vi "ParseTXT.vi"(8 "error in (no error)":errorcluster, 10 "Path":path=path "C:/LVLibrary/XNET/XCP_DaqDtoID/XCP_DaqDtoId/ECUMCLog/XCP or CCP Master_Protocol_Log.txt", 11 "DAQList in":refnum<class "DAQList.lvclass">) -> (0 "error out":errorcluster, 2 "CAN Frames":T1[](array[typedef])=[{"timestamp"=timestamp(0 s since 1904-01-01), "payload"=[255, 0, 109, 101, 0, 39, 0, 0, 0], "identifier"=1996, "type"=0, "extended?"=FALSE, "echo?"=FALSE}, {"timestamp"=timestamp(0 s since 1904-01-01), "payload"=[253, 255, 255, 255, 0, 0, 0, 0, 0], "identifier"=1996, "type"=0, "extended?"=FALSE, "echo?"=FALSE}, {"timestamp"=timestamp(0 s since 1904-01-01), "payload"=[251, 255, 255, 255, 0, 0, 0, 0, 0], "identifier"=1996, "type"=0, "extended?"=FALSE, "echo?"=FALSE}, {"timestamp"=timestamp(0 s since 1904-01-01), "payload"=[218, 120, 84, 83, 83, 0, 0, 0, 0], "identifier"=1996, "type"=0, "extended?"=FALSE, "echo?"=FALSE}, {"timestamp"=timestamp(0 s since 1904-01-01), "payload"=[215, 0, 0, 0, 66, 0, 0, 0, 0], "identifier"=1996, "type"=0, "extended?"=FALSE, "echo?"=FALSE}, {"timestamp"=timestamp(0 s since 1904-01-01), "payload"=[245, 7, 114, 76, 101, 110, 0, 0, 0], "identifier"=1996, "type"=0, "extended?"=FALSE, "echo?"=FALSE}, {"timestamp"=timestamp(0 s since 1904-01-01), "payload"=[245, 7, 114, 76, 101, 110, 0, 0, 0], "identifier"=1996, "type"=0, "extended?"=FALSE, "echo?"=FALSE}, {"timestamp"=timestamp(0 s since 1904-01-01), "payload"=[245, 5, 114, 76, 101, 110, 0, 0, 0], "identifier"=1996, "type"=0, "extended?"=FALSE, "echo?"=FALSE}, {"timestamp"=timestamp(0 s since 1904-01-01), "payload"=[215, 0, 0, 0, 0, 0, 0, 0, 0], "identifier"=1996, "type"=0, "extended?"=FALSE, "echo?"=FALSE}, {"timestamp"=timestamp(0 s since 1904-01-01), "payload"=[245, 7, 66, 105, 116, 0, 0, 0, 0], "identifier"=1996, "type"=0, "extended?"=FALSE, "echo?"=FALSE}, {"timestamp"=timestamp(0 s since 1904-01-01), "payload"=[245, 7, 66, 105, 116, 0, 0, 0, 0], "identifier"=1996, "type"=0, "extended?"=FALSE, "echo?"=FALSE}, {"timestamp"=timestamp(0 s since 1904-01-01), "payload"=[245, 5, 66, 105, 116, 0, 0, 0, 0], "identifier"=1996, "type"=0, "extended?"=FALSE, "echo?"=FALSE}, {"timestamp"=timestamp(0 s since 1904-01-01), "payload"=[215, 0, 1, 0, 101, 0, 0, 0, 0], "identifier"=1996, "type"=0, "extended?"=FALSE, "echo?"=FALSE}, {"timestamp"=timestamp(0 s since 1904-01-01), "payload"=[245, 7, 114, 105, 103, 115, 0, 0, 0], "identifier"=1996, "type"=0, "extended?"=FALSE, "echo?"=FALSE}, {"timestamp"=timestamp(0 s since 1904-01-01), "payload"=[245, 7, 114, 105, 103, 115, 0, 0, 0], "identifier"=1996, "type"=0, "extended?"=FALSE, "echo?"=FALSE}, {"timestamp"=timestamp(0 s since 1904-01-01), "payload"=[245, 6, 114, 105, 103, 115, 0, 0, 0], "identifier"=1996, "type"=0, "extended?"=FALSE, "echo?"=FALSE}, {"timestamp"=timestamp(0 s since 1904-01-01), "payload"=[215, 0, 2, 0, 109, 101, 0, 0, 0], "identifier"=1996, "type"=0, "extended?"=FALSE, "echo?"=FALSE}, {"timestamp"=timestamp(0 s since 1904-01-01), "payload"=[245, 7, 0, 0, 66, 0, 0, 0, 0], "identifier"=1996, "type"=0, "extended?"=FALSE, "echo?"=FALSE}, {"timestamp"=timestamp(0 s since 1904-01-01), "payload"=[245, 7, 0, 0, 66, 0, 0, 0, 0], "identifier"=1996, "type"=0, "extended?"=FALSE, "echo?"=FALSE}, {"timestamp"=timestamp(0 s since 1904-01-01), "payload"=[245, 6, 0, 0, 66, 0, 0, 0, 0], "identifier"=1996, "type"=0, "extended?"=FALSE, "echo?"=FALSE}, {"timestamp"=timestamp(0 s since 1904-01-01), "payload"=[215, 0, 3, 0, 0, 39, 0, 0, 0], "identifier"=1996, "type"=0, "extended?"=FALSE, "echo?"=FALSE}, {"timestamp"=timestamp(0 s since 1904-01-01), "payload"=[245, 7, 84, 83, 83, 0, 0, 0, 0], "identifier"=1996, "type"=0, "extended?"=FALSE, "echo?"=FALSE}, {"timestamp"=timestamp(0 s since 1904-01-01), "payload"=[245, 7, 84, 83, 83, 0, 0, 0, 0], "identifier"=1996, "type"=0, "extended?"=FALSE, "echo?"=FALSE}, {"timestamp"=timestamp(0 s since 1904-01-01), "payload"=[245, 7, 84, 83, 83, 0, 0, 0, 0], "identifier"=1996, "type"=0, "extended?"=FALSE, "echo?"=FALSE}, {"timestamp"=timestamp(0 s since 1904-01-01), "payload"=[215, 0, 4, 0, 66, 0, 0, 0, 0], "identifier"=1996, "type"=0, "extended?"=FALSE, "echo?"=FALSE}, {"timestamp"=timestamp(0 s since 1904-01-01), "payload"=[245, 7, 67, 121, 99, 108, 101, 0, 0], "identifier"=1996, "type"=0, "extended?"=FALSE, "echo?"=FALSE}, {"timestamp"=timestamp(0 s since 1904-01-01), "payload"=[245, 7, 67, 121, 99, 108, 101, 0, 0], "identifier"=1996, "type"=0, "extended?"=FALSE, "echo?"=FALSE}, {"timestamp"=timestamp(0 s since 1904-01-01), "payload"=[245, 7, 67, 121, 99, 108, 101, 0, 0], "identifier"=1996, "type"=0, "extended?"=FALSE, "echo?"=FALSE}, {"timestamp"=timestamp(0 s since 1904-01-01), "payload"=[245, 1, 67, 121, 99, 108, 101, 0, 0], "identifier"=1996, "type"=0, "extended?"=FALSE, "echo?"=FALSE}, {"timestamp"=timestamp(0 s since 1904-01-01), "payload"=[217, 255, 255, 255, 0, 0, 0, 0, 0], "identifier"=1996, "type"=0, "extended?"=FALSE, "echo?"=FALSE}, {"timestamp"=timestamp(0 s since 1904-01-01), "payload"=[233, 255, 255, 255, 0, 0, 0, 0, 0], "identifier"=1996, "type"=0, "extended?"=FALSE, "echo?"=FALSE}, {"timestamp"=timestamp(0 s since 1904-01-01), "payload"=[232, 0, 0, 0, 0, 108, 101, 0, 0], "identifier"=1996, "type"=0, "extended?"=FALSE, "echo?"=FALSE}, {"timestamp"=timestamp(0 s since 1904-01-01), "payload"=[232, 0, 0, 1, 0, 108, 101, 0, 0], "identifier"=1996, "type"=0, "extended?"=FALSE, "echo?"=FALSE}, {"timestamp"=timestamp(0 s since 1904-01-01), "payload"=[232, 1, 0, 1, 0, 108, 101, 0, 0], "identifier"=1996, "type"=0, "extended?"=FALSE, "echo?"=FALSE}, {"timestamp"=timestamp(0 s since 1904-01-01), "payload"=[231, 0, 0, 0, 101, 0, 0, 0, 0], "identifier"=1996, "type"=0, "extended?"=FALSE, "echo?"=FALSE}, {"timestamp"=timestamp(0 s since 1904-01-01), "payload"=[206, 255, 255, 255, 0, 0, 0, 0, 0], "identifier"=1996, "type"=0, "extended?"=FALSE, "echo?"=FALSE}, {"timestamp"=timestamp(0 s since 1904-01-01), "payload"=[227, 0, 0, 0, 0, 2, 0, 0, 0], "identifier"=1996, "type"=0, "extended?"=FALSE, "echo?"=FALSE}, {"timestamp"=timestamp(0 s since 1904-01-01), "payload"=[226, 0, 0, 0, 0, 0, 0, 0, 0], "identifier"=1996, "type"=0, "extended?"=FALSE, "echo?"=FALSE}, {"timestamp"=timestamp(0 s since 1904-01-01), "payload"=[225, 255, 1, 0, 112, 172, 0, 80, 0], "identifier"=1996, "type"=0, "extended?"=FALSE, "echo?"=FALSE}, {"timestamp"=timestamp(0 s since 1904-01-01), "payload"=[225, 255, 1, 0, 113, 172, 0, 80, 0], "identifier"=1996, "type"=0, "extended?"=FALSE, "echo?"=FALSE}, {"timestamp"=timestamp(0 s since 1904-01-01), "payload"=[225, 255, 1, 0, 114, 172, 0, 80, 0], "identifier"=1996, "type"=0, "extended?"=FALSE, "echo?"=FALSE}, {"timestamp"=timestamp(0 s since 1904-01-01), "payload"=[225, 255, 1, 0, 115, 172, 0, 80, 0], "identifier"=1996, "type"=0, "extended?"=FALSE, "echo?"=FALSE}, {"timestamp"=timestamp(0 s since 1904-01-01), "payload"=[224, 0, 0, 0, 0, 0, 1, 0, 0], "identifier"=1996, "type"=0, "extended?"=FALSE, "echo?"=FALSE}, {"timestamp"=timestamp(0 s since 1904-01-01), "payload"=[222, 2, 0, 0, 0, 39, 0, 0, 0], "identifier"=1996, "type"=0, "extended?"=FALSE, "echo?"=FALSE}, {"timestamp"=timestamp(0 s since 1904-01-01), "payload"=[254, 54, 78, 51, 35, 2, 0, 0, 0], "identifier"=1996, "type"=0, "extended?"=FALSE, "echo?"=FALSE}] {"payload" format="%x"; "timestamp" format="%<%.7X\n%x>T"; "type" items=["CAN Data"=0, "CAN Remote"=1, "CAN Bus Error"=2, "CAN 2.0 Data"=8, "CAN FD Data"=16, "CAN FD+BRS Data"=24, "J1939 Data"=192, "Delay"=224, "Log Trigger"=225, "Start Trigger"=226]; "identifier" format="%x"}, 3 "DAQList out":refnum<class "DAQList.lvclass">)   [LabVIEW 2019, in "XCP_DaqDtoId.lvlib" / "DAQList.lvclass"]
uses:
  DAQList.lvclass
  <vilib>/xnet/xnet.llb/XNET Frame CAN.ctl
  <vilib>/xnet/xnet.llb/XNET Frame Type CAN.ctl
  DAQList.lvclass/DAQList.ctl
  <vilib>/Utility/file.llb/Read Delimited Spreadsheet (string).vi
  <vilib>/ECUMC/ECUMC.llb/MC Get Prop XCP CRO Id.vi
  <vilib>/ECUMC/ECUMC.llb/MC Get Prop XCP DTO Id.vi
  <vilib>/ECUMC/ECUMC.lvlib
panel:
  in  "Debug Mode":bool
  in  "IDs (debug only)":u32[](array[numeric]) format="%.0x"
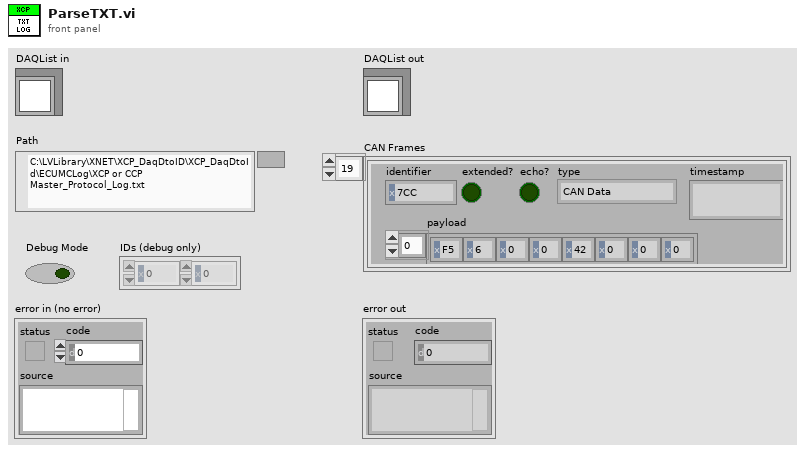
[diagram p1: front panel]
types:
  T1 = typedef "XNET Frame CAN.ctl" = cluster{"timestamp":timestamp, "payload":u8[], "identifier":u32, "type":T2, "extended?":bool, "echo?":bool}
  T2 = typedef "XNET Frame Type CAN.ctl" = u8
  T3 = typedef "ECUMC.lvlib/MC Reference.ctt" = u32
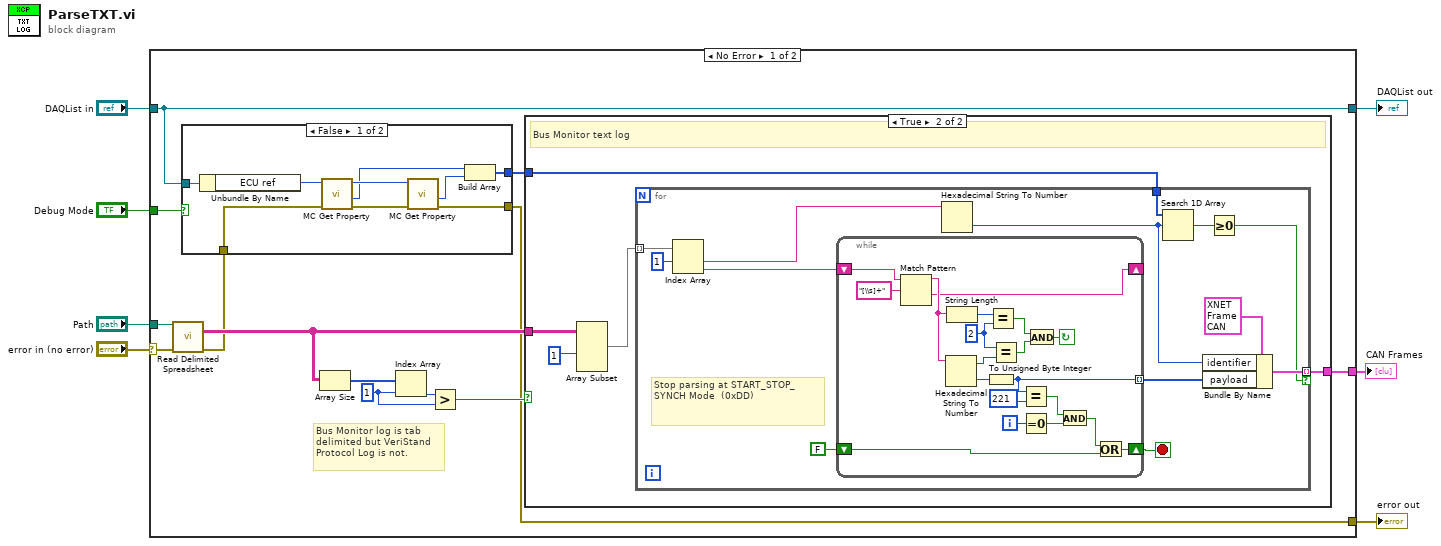
[diagram p0: block diagram]
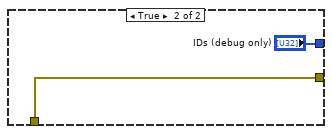
[diagram p2: hidden frame]
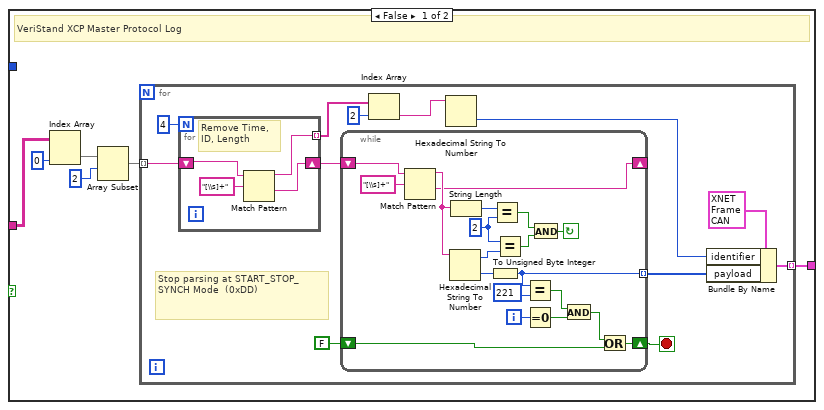
[diagram p3: hidden frame]
diagram:
  n1 = case shown="No Error" "error in (no error)" {
    selector: "error in (no error)" -> [w19 w111]
    tunnel: [w10 w111] -> w6
    tunnel: [w12 w110] -> w4
    tunnel: "DAQList in" -> [w12 w110]
    tunnel: "Path" -> [w20 _]
    tunnel: [w18 _] -> w2
    tunnel: "Debug Mode" -> [w8 _]
    frame No Error {
      w14 = 1 ("index")
      # "Bus Monitor log is tab delimited but VeriStand Protocol Log is not."
      n2 = call-poly <vilib>:"Read Delimited Spreadsheet.vi"("file path (dialog if empty)"=w20, "error in (no error)"=w19) -> ("all rows"=w17:string[][], "error out"=w11:errorcluster)  [unwired: 8 in, 4 out]
      n3 = case shown="False" w8 {
        tunnel: w12 -> [w29 _]
        tunnel: w11 -> [w27 w31]
        tunnel: [w24 w31] -> w10
        tunnel: [w21 "IDs (debug only)"] -> w9
        frame False {
          n4 = Unbundle By Name(w29) -> ("ECU ref"=w28:T3)
          n5 = call-poly <vilib>:"MC Get Property.vi"("error in"=w27, "reference in"=w28) -> ("error out"=w25:errorcluster, "XCP CRO id"=w23:u32, "reference out"=w26:T3)  [unwired: 7 in]
          n6 = call-poly <vilib>:"MC Get Property.vi"("error in"=w25, "reference in"=w26) -> ("error out"=w24:errorcluster, "XCP DTO id"=w22:u32)  [unwired: 7 in, 1 out]
          n7 = Build Array(w23, w22) -> (w21:u32[])
        }
        frame True {
        }
      }
      n8 = Array Size(array=w17) -> (size(s)=w16:i32[])
      n9 = Index Array(array=w16, index=w14) -> (element=w15:i32)
      n10 = Greater?(x=w15, y=w14) -> (0:w13:bool)
      n11 = case shown="True" w13 {
        tunnel: [w33 w74] -> w18
        tunnel: w17 -> [w32 w75]
        tunnel: w9 -> [_ w73]
        frame False {
          # "VeriStand XCP Master Protocol Log"
          n12 = Index Array(array=w32, index (col)=0 ("disabled index (col)")) -> (element=w35:string[])  [unwired: 1 in]
          n13 = Array Subset(array=w35, index=2) -> (w34:string[])  [unwired: 1 in]
          n14 = for {
            tunnel: w34 -> [w45] mode=indexing
            tunnel: [w44] -> w33 mode=indexing
            stop <- w38 stop-if-true
            # "Stop parsing at START_STOP_SYNCH Mode  (0xDD)"
            n15 = for {
              N: 4 -> [_]
              shift-right: [w70] -> w48
              shift-left: w45 -> [w72]
              tunnel: [w69] -> w43 mode=indexing
              # "Remove Time, ID, Length"
              n16 = Match Pattern(string=w72, regular expression="[\\s]+") -> (before substring=w69:string, after substring=w70:string)  [unwired: 1 in, 2 out]
            }
            n17 = while {
              shift-right: [w59] -> _
              shift-left: w48 -> [w68]
              tunnel: [w56] -> w46 mode=indexing
              shift-right: [w51] -> w38
              shift-left: FALSE -> [w50]
              i -> [w57]
              stop <- w60 continue-if-true
              w64 = 2 ("y")
              n18 = Match Pattern(string=w68, regular expression="[\\s]+") -> (before substring=w65:string, after substring=w59:string)  [unwired: 1 in, 2 out]
              n19 = Hexadecimal String To Number(string=w65) -> (offset past number=w63:i32, number=w58:u32)  [unwired: 2 in]
              n20 = String Length(string=w65) -> (length=w66:i32)
              n21 = To Unsigned Byte Integer(number=w58) -> (unsigned 8bit integer=w56:u8)
              n22 = Equal?(x=w66, y=w64) -> (x = y?=w62:bool)
              n23 = Equal?(x=w64, y=w63) -> (x = y?=w61:bool)
              n24 = Equal?(x=w56, y=u8 221 ("unsigned 8bit integer")) -> (x = y?=w54:bool)
              n25 = Equal To 0?(x=w57) -> (x = 0?=w53:bool)
              n26 = And(x=w62, y=w61) -> (x .and. y?=w60:bool)
              n27 = And(x=w54, y=w53) -> (x .and. y?=w52:bool)
              n28 = Or(x=w52, y=w50) -> (x .or. y?=w51:bool)
            }
            n29 = Index Array(array=w43, index=2) -> (element=w41:string)
            n30 = Hexadecimal String To Number(string=w41) -> (number=w40:u32)  [unwired: 2 in, 1 out]
            n31 = Bundle By Name(cluster=T1 {"timestamp"=timestamp(0 s since 1904-01-01), "payload"=[], "identifier"=0, "type"=0, "extended?"=FALSE, "echo?"=FALSE} ("CAN frame"), "identifier"=w40, "payload"=w46) -> (w44:T1)
          }
        }
        frame True {
          # "Bus Monitor text log"
          n32 = Array Subset(array=w75, index (row)=1 ("index")) -> (w76:string[][])  [unwired: 3 in]
          n33 = for {
            tunnel: w76 -> [w83] mode=indexing
            tunnel: [w88] -> w74 mode=indexing if=w78
            tunnel: w73 -> [w81]
            stop <- w84 stop-if-true
            # "Stop parsing at START_STOP_SYNCH Mode  (0xDD)"
            n34 = Index Array(array=w83, index #1=1 ("index")) -> (element #1=w86:string, element #2=w82:string)  [unwired: 1 in]
            n35 = while {
              shift-right: [w100] -> _
              shift-left: w82 -> [w109]
              tunnel: [w97] -> w89 mode=indexing
              shift-right: [w92] -> w84
              shift-left: FALSE -> [w91]
              i -> [w98]
              stop <- w101 continue-if-true
              w105 = 2 ("y")
              n36 = Match Pattern(string=w109, regular expression="[\\s]+") -> (before substring=w106:string, after substring=w100:string)  [unwired: 1 in, 2 out]
              n37 = Hexadecimal String To Number(string=w106) -> (offset past number=w104:i32, number=w99:u32)  [unwired: 2 in]
              n38 = String Length(string=w106) -> (length=w107:i32)
              n39 = To Unsigned Byte Integer(number=w99) -> (unsigned 8bit integer=w97:u8)
              n40 = Equal?(x=w107, y=w105) -> (x = y?=w103:bool)
              n41 = Equal?(x=w105, y=w104) -> (x = y?=w102:bool)
              n42 = Equal?(x=w97, y=u8 221 ("unsigned 8bit integer")) -> (x = y?=w95:bool)
              n43 = Equal To 0?(x=w98) -> (x = 0?=w94:bool)
              n44 = And(x=w103, y=w102) -> (x .and. y?=w101:bool)
              n45 = And(x=w95, y=w94) -> (x .and. y?=w93:bool)
              n46 = Or(x=w93, y=w91) -> (x .or. y?=w92:bool)
            }
            n47 = Hexadecimal String To Number(string=w86) -> (number=w80:u32)  [unwired: 2 in, 1 out]
            n48 = Search 1D Array(1D array=w81, element=w80) -> (index of element=w79:i32)  [unwired: 1 in]
            n49 = Bundle By Name(cluster=T1 {"timestamp"=timestamp(0 s since 1904-01-01), "payload"=[], "identifier"=0, "type"=0, "extended?"=FALSE, "echo?"=FALSE} ("CAN frame"), "identifier"=w80, "payload"=w89) -> (w88:T1)
            n50 = Greater Or Equal To 0?(x=w79) -> (x >= 0?=w78:bool)
          }
        }
      }
    }
    frame Error {
    }
  }
  "error out" <- w6
  "DAQList out" <- w4
  "CAN Frames" <- w2
